vi "Pneumatics_Monitor.vi"(8 "error in":errorcluster) -> (0 "error out":errorcluster)   [LabVIEW 2020]
uses:
  <vilib>/Rock Robotics/Network Tables/NT Write Boolean.vi
  <vilib>/Rock Robotics/Network Tables/NT Write Number.vi
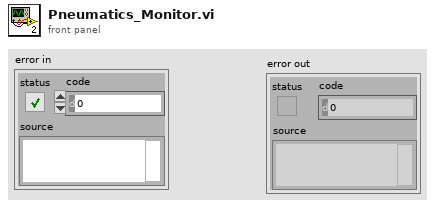
[diagram p1: front panel]
types:
  T1 = typedef "WPI_CompressorDevRef.ctl" = cluster{"DevStatus":errorcluster, "Pneumatics Control Module":u8}
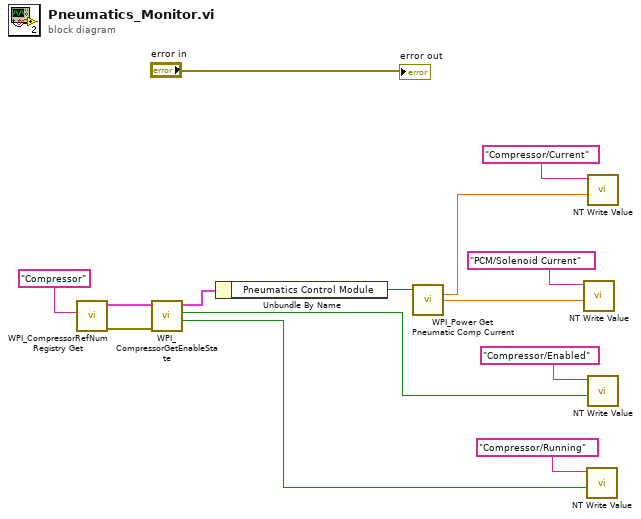
[diagram p0: block diagram]
diagram:
  n1 = call <vilib>:"WPI_CompressorRefNum Registry Get.vi"("refnum name"="Compressor") -> ("error out"=w11:errorcluster, "CompressorDevRef"=w12:T1)  [unwired: 9 in]
  n2 = call <vilib>:"WPI_CompressorGetEnableState.vi"("error in (no error)"=w11, "CompressorDevRef"=w12) -> ("Compressor Running"=w6:bool, "Enabled"=w5:bool, "CompressorDevRef"=w10:T1)  [unwired: 3 in, 4 out]
  n3 = Unbundle By Name(w10) -> ("Pneumatics Control Module"=w9:u8)
  n4 = call <vilib>:"WPI_Power Get Pneumatic Comp Current.vi"("Pneumatics device (def)"=w9) -> ("current (A)"=w2:dbl, "Total Solenoid A"=w1:dbl)  [unwired: 12 in, 1 out]
  n5 = call-poly <vilib>:"NT Write Value.vi"("value"=w1, "name"="PCM/Solenoid Current") -> ()  [unwired: 9 in, 1 out]
  n6 = call-poly <vilib>:"NT Write Value.vi"("value"=w6, "name"="Compressor/Running") -> ()  [unwired: 9 in, 1 out]
  n7 = call-poly <vilib>:"NT Write Value.vi"("value"=w2, "name"="Compressor/Current") -> ()  [unwired: 9 in, 1 out]
  n8 = call-poly <vilib>:"NT Write Value.vi"("value"=w5, "name"="Compressor/Enabled") -> ()  [unwired: 9 in, 1 out]
  "error out" <- "error in"
